vi "Maintenance.vi"() -> ()   [LabVIEW 2020, in "Maintenance Lib.lvlib"]
uses:
  Maintenance Lib.lvlib
  Database Lib.lvlib
panel:
  in  "Close":bool
  out "Table Control":string[][](table)
  # "Maintenance"
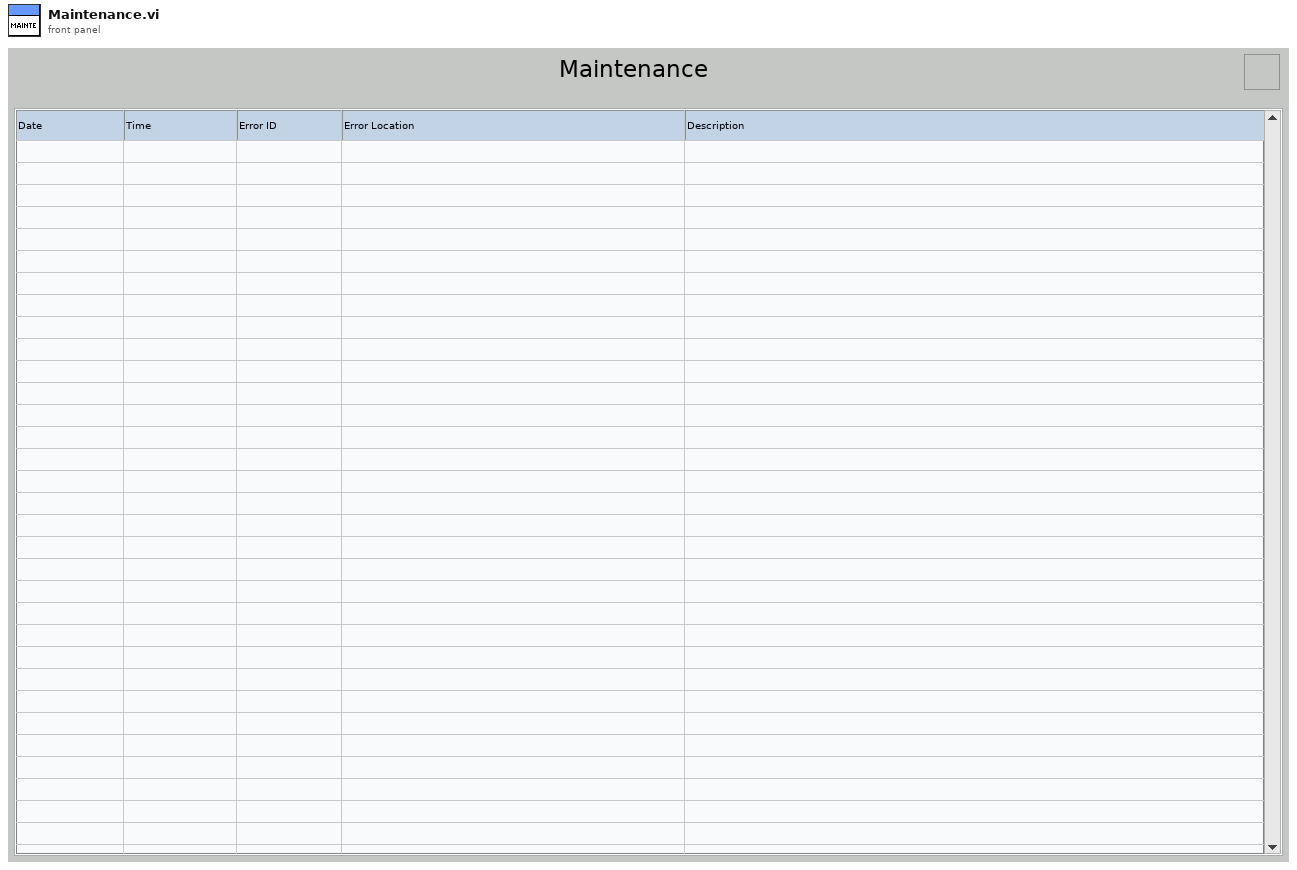
[diagram p1: front panel]
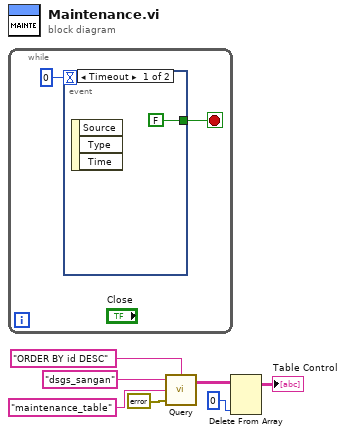
[diagram p0: block diagram]
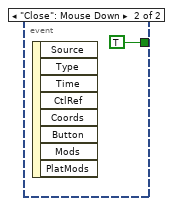
[diagram p2: hidden frame]
diagram:
  n1 = while {
    stop <- w9 stop-if-true
    n2 = event shown="[0] Timeout" {
      selector: _ -> [_ _]
      dyn-events: _ -> [_ _]
      timeout: 0 -> [_ _]
      tunnel: [FALSE TRUE] -> w9
      event Timeout {
        n3 = event-data() -> ()  [unwired: 1 in, 3 out]
      }
      event "Close": Mouse Down {
        n4 = event-data() -> ()  [unwired: 1 in, 8 out]
      }
    }
  }
  n5 = call "Query.vi"("Condition"="ORDER BY id DESC", "Error in"=errorcluster {"status"=FALSE, "code"=0, "source"=""}, "Table Name"="maintenance_table", "Connection Name"="dsgs_sangan") -> ("data"=w4:string[][])  [unwired: 1 out]
  n6 = Delete From Array(array=w4, index (col)=0 ("disabled index (col)")) -> (array with subset deleted=→"Table Control":string[][])  [unwired: 2 in, 1 out]
